vi "ImportXML.vi"(8 "error in (no error)":errorcluster, 10 "selected path":path=path "C:/Users/tq7638/Desktop/hjghg.xml", 11 "Node Ptr":T1 format="%.0x") -> (0 "error out":errorcluster, 3 "Node Ptr Out":T1 format="%.0x")   [LabVIEW 2024, in "Embedded TDMS Logger System Explorer.lvlib"]
doc: "Import the configuration of the Custom Device from an XML file."
uses:
  Embedded TDMS Logger System Explorer.lvlib
  <vilib>/NI VeriStand/Custom Device API/Custom Device Item Ref.ctl
  Shared/File Classes/File/FileAsCluster.ctl
  Shared/File Classes/Group/GroupAsCluster.ctl
  Shared/File Classes/Channel/ChannelAsCluster.ctl
  <vilib>/NI VeriStand/Custom Device API/Data Reference.ctl
  Shared/File Classes/Meta Data.ctl
  Shared/Segmentation.ctl
  Shared/SegmentOptions.ctl
  <vilib>/NI VeriStand/Custom Device API/Set Item Property (Boolean).vi
  <vilib>/NI VeriStand/Custom Device API/Set Item Property (Double).vi
  <vilib>/NI VeriStand/Custom Device API/Set Item Property (U16).vi
  <vilib>/regexp/Match Regular Expression.xnode
  <vilib>/NI VeriStand/Custom Device API/Custom Device API.lvlib
  Shared/File Classes/File/File.lvclass
  Shared/Embedded TDMS Logger Shared.lvlib
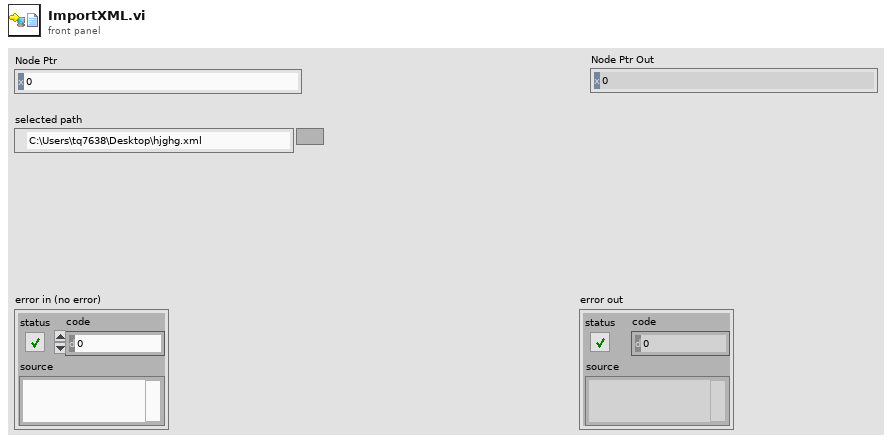
[diagram p1: front panel]
types:
  T1 = typedef "Custom Device API.lvlib/Custom Device Item Ref.ctl" = u64
  T2 = typedef "Embedded TDMS Logger Shared.lvlib/Segmentation.ctl" = cluster{"Segment":bool, "Segment Every":dbl, "Segment by":T3}
  T3 = typedef "SegmentOptions.ctl" = enum16{"Time (s)", "Size (MB)"}
  T4 = typedef "FileAsCluster.ctl" = cluster{"Name":string, "Directory":string, "Date Captured":string, "Groups":T5[], "Meta Data":T8[], "File Start Time":timestamp, "appended path":path}
  T5 = typedef "GroupAsCluster.ctl" = cluster{"Name":string, "Channels":T6[], "Meta Data":T8[]}
  T6 = typedef "ChannelAsCluster.ctl" = cluster{"Name":string, "Data Reference":T7, "Wfm?":bool, "Decimation":i32, "Current Value":dbl, "Meta Data":T8[], "WfmPath":string}
  T7 = typedef "Custom Device API.lvlib/Data Reference.ctl" = i32
  T8 = typedef "Meta Data.ctl" = cluster{"Key":string, "Value":string}
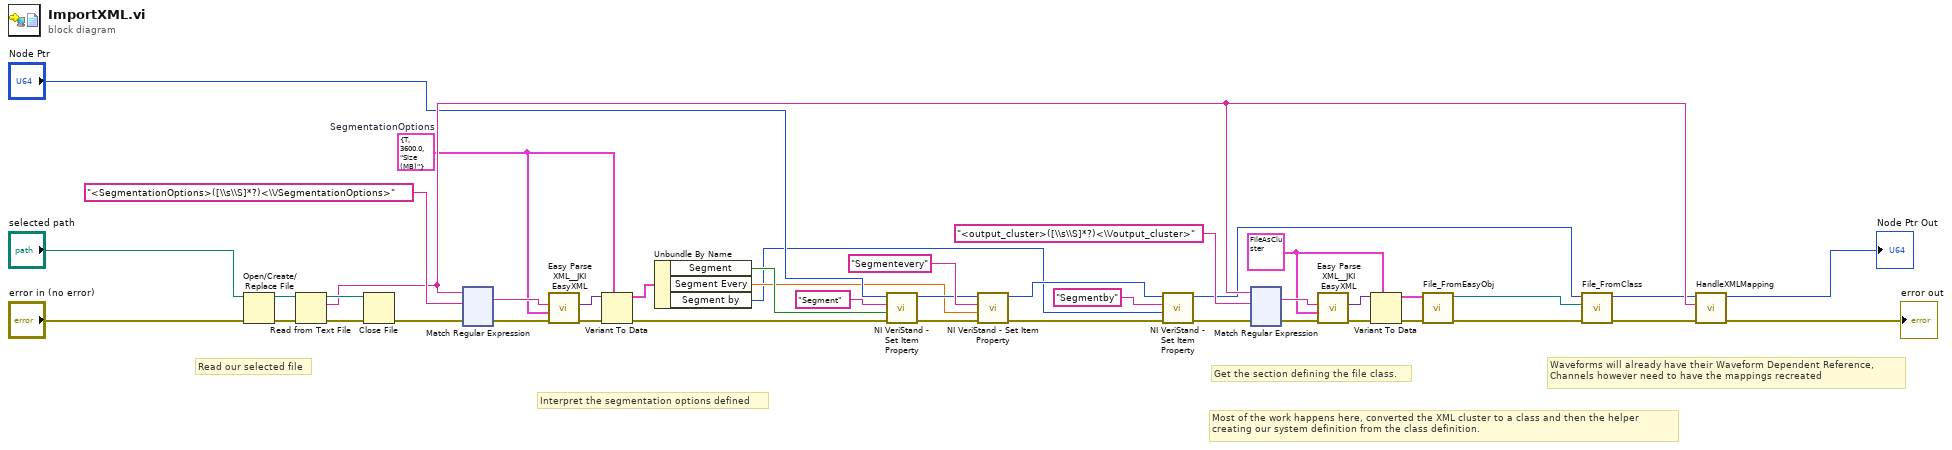
[diagram p0: block diagram]
diagram:
  w21 = T2 {"Segment"=TRUE, "Segment Every"=3600.0, "Segment by"=enum."Size (MB)"}  # SegmentationOptions
  w36 = T4 {"Name"="", "Directory"="", "Date Captured"="", "Groups"=[], "Meta Data"=[], "File Start Time"=timestamp(0 s since 1904-01-01), "appended path"=path ""} ("output cluster")
  # "Most of the work happens here, converted the XML cluster to a class and then the helper\ncreating our system definition from the class definition."
  # "Interpret the segmentation options defined"
  # "Get the section defining the file class."
  # "Read our selected file"
  # "Waveforms will already have their Waveform Dependent Reference,\nChannels however need to have the mappings recreated"
  n1 = Open/Create/Replace File(file path (use dialog)="selected path", error in="error in (no error)") -> (refnum out=w34:refnum<file>, error out=w33:errorcluster)  [unwired: 4 in, 1 out]
  n2 = Read from Text File(file (use dialog)=w34, error in=w33) -> (refnum out=w42:refnum<file>, text=w25:string, error out=w41:errorcluster)  [unwired: 2 in, 1 out]
  n3 = Close File(refnum=w42, error in=w41) -> (error out=w2:errorcluster)  [unwired: 1 out]
  n4 = xnode "Match Regular Expression"("input string"=w25, "regular expression"="<SegmentationOptions>([\\s\\S]*?)<\\/SegmentationOptions>" ("format string"), "error in"=w2) -> ("whole match"=w24:string, "error out"=w23:errorcluster)  [unwired: 3 in, 3 out]
  n5 = call <vilib>:"Easy Parse XML__JKI EasyXML.vi"("error in (no error)"=w23, "LabVIEW Data (Type)"=w21, "XML String"=w24) -> ("error out"=w20:errorcluster, "LabVIEW Data"=w22:variant)  [unwired: 7 in]
  n6 = Variant To Data(error in=w20, type=w21, Variant=w22) -> (data=w12:T2, error out=w6:errorcluster)
  n7 = Unbundle By Name(w12) -> ("Segment"=w11:bool, "Segment Every"=w10:dbl, "Segment by"=w9:T3)
  n8 = call-poly <vilib>:"NI VeriStand - Set Item Property.vi"("error in (no error)"=w6, "Value"=w11, "Property Name"="Segment", "Item Ref in"="Node Ptr") -> ("error out"=w7:errorcluster, "Item Ref out"=w15:T1)  [unwired: 5 in, 1 out]
  n9 = call-poly <vilib>:"NI VeriStand - Set Item Property.vi"("error in (no error)"=w7, "Value"=w10, "Property Name"="Segmentevery", "Item Ref in"=w15) -> ("error out"=w8:errorcluster, "Item Ref out"=w14:T1)  [unwired: 5 in, 1 out]
  n10 = call-poly <vilib>:"NI VeriStand - Set Item Property.vi"("error in (no error)"=w8, "Value"=w9, "Property Name"="Segmentby", "Item Ref in"=w14) -> ("error out"=w1:errorcluster, "Item Ref out"=w13:T1)  [unwired: 5 in, 1 out]
  n11 = xnode "Match Regular Expression"("input string"=w25, "regular expression"="<output_cluster>([\\s\\S]*?)<\\/output_cluster>" ("format string"), "error in"=w1) -> ("whole match"=w39:string, "error out"=w3:errorcluster)  [unwired: 3 in, 3 out]
  n12 = call <vilib>:"Easy Parse XML__JKI EasyXML.vi"("error in (no error)"=w3, "LabVIEW Data (Type)"=w36, "XML String"=w39) -> ("error out"=w38:errorcluster, "LabVIEW Data"=w37:variant)  [unwired: 7 in]
  n13 = Variant To Data(error in=w38, type=w36, Variant=w37) -> (data=w35:T4, error out=w31:errorcluster)
  n14 = call "File_FromEasyObj.vi"("error in (no error)"=w31, "output cluster"=w35) -> ("error out"=w29:errorcluster, "File out"=w30:refnum<class "File.lvclass">)  [unwired: 8 in]
  n15 = call "File_FromClass.vi"("error in (no error)"=w29, "File.lvclass"=w30, "Node Ptr"=w13) -> ("error out"=w28:errorcluster, "Node Ptr Out"=w4:T1)  [unwired: 7 in]
  n16 = call "HandleXMLMapping.vi"("error in (no error)"=w28, "String"=w25, "Node Ptr"=w4) -> ("error out"=→"error out":errorcluster, "Node Ptr Out"=→"Node Ptr Out":T1)  [unwired: 7 in]
